vi "CS POLARIS BME DG.Delete DIMServices.vi"(8 "error in (no error)":errorcluster, 11 "BME_DG_System in":refnum<class "BME_DG_System.lvclass">) -> (0 "error out":errorcluster, 3 "BME_DG_System out":refnum<class "BME_DG_System.lvclass">)   [LabVIEW 2009, in "CS POLARIS BME DG.lvlib"]
uses:
  CS POLARIS BME DG.lvlib
  DG Classes/BME_DG_System/BME_DG_System.lvclass
  DG Classes/BME_DG_Base/BME_DG_Base.lvclass
  DG Classes/BME_DG_Chnl/BME_DG_Chnl.lvclass
  lib.lib/DimLVEvent/LVDimInterface/LVDimInterface.lvlib
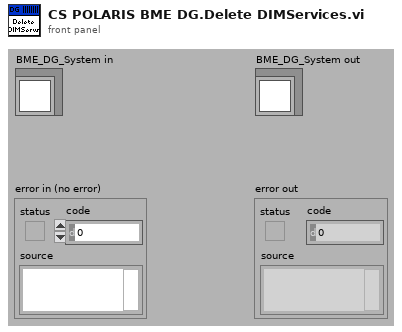
[diagram p1: front panel]
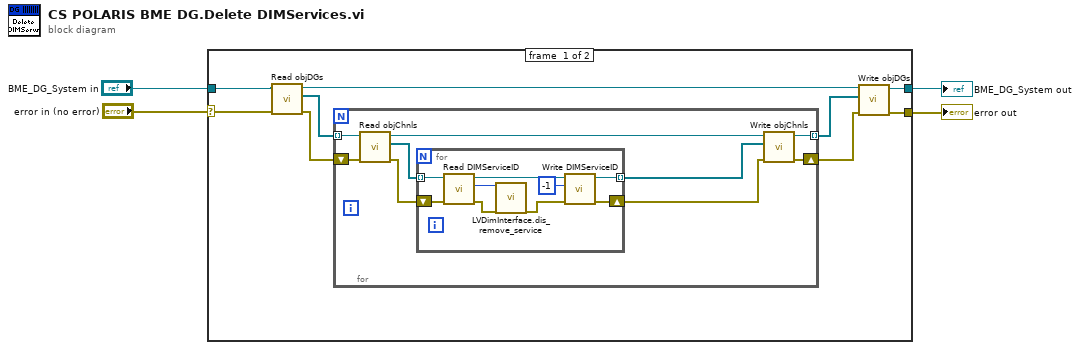
[diagram p0: block diagram]
diagram:
  n1 = case shown="No Error" "error in (no error)" {
    selector: "error in (no error)" -> [w12 w33]
    tunnel: [w5 w33] -> w3
    tunnel: "BME_DG_System in" -> [w13 w32]
    tunnel: [w9 w32] -> w1
    frame #0 {
      n2 = call "Read objDGs.vi"("error in (no error)"=w12, "BME_DG_System in"=w13) -> ("error out"=w7:errorcluster, "objDGs"=w11:refnum<class "BME_DG_Base.lvclass">[], "BME_DG_System out"=w10:refnum<class "BME_DG_System.lvclass">)  [unwired: 7 in]
      n3 = for {
        tunnel: w11 -> [w22] mode=indexing
        tunnel: [w20] -> w8 mode=indexing
        shift-right: [w16] -> w6
        shift-left: w7 -> [w15]
        n4 = call-dynamic "Read objChnls.vi"("error in (no error)"=w15, "BME_DG_Base in"=w22) -> ("error out"=w18:errorcluster, "objChnls"=w19:refnum<class "BME_DG_Chnl.lvclass">[], "BME_DG_Base out"=w21:refnum<class "BME_DG_Base.lvclass">)  [unwired: 6 in, 1 out]
        n5 = for {
          tunnel: w19 -> [w23] mode=indexing
          tunnel: [w31] -> w17 mode=indexing
          shift-right: [w30] -> w14
          shift-left: w18 -> [w24]
          n6 = call-dynamic "Read DIMServiceID.vi"("error in (no error)"=w24, "BME_DG_Chnl in"=w23) -> ("error out"=w27:errorcluster, "DIMServiceID"=w26:i32, "BME_DG_Chnl out"=w28:refnum<class "BME_DG_Chnl.lvclass">)  [unwired: 7 in]
          n7 = call "LVDimInterface.dis_remove_service.vi"("my_serviceID"=w26, "error in (no error)"=w27) -> ("error out"=w29:errorcluster)  [unwired: 17 in]
          n8 = call-dynamic "Write DIMServiceID.vi"("error in (no error)"=w29, "DIMServiceID"=-1, "BME_DG_Chnl in"=w28) -> ("error out"=w30:errorcluster, "BME_DG_Chnl out"=w31:refnum<class "BME_DG_Chnl.lvclass">)  [unwired: 7 in]
        }
        n9 = call-dynamic "Write objChnls.vi"("error in (no error)"=w14, "objChnls"=w17, "BME_DG_Base in"=w21) -> ("error out"=w16:errorcluster, "BME_DG_Base out"=w20:refnum<class "BME_DG_Base.lvclass">)  [unwired: 7 in]
      }
      n10 = call "Write objDGs.vi"("error in (no error)"=w6, "objDGs"=w8, "BME_DG_System in"=w10) -> ("error out"=w5:errorcluster, "BME_DG_System out"=w9:refnum<class "BME_DG_System.lvclass">)  [unwired: 7 in]
    }
    frame #1 {
    }
  }
  "error out" <- w3
  "BME_DG_System out" <- w1
